vi "Write Last Temperature.vi"(8 "error in (no error)":errorcluster, 10 "Last Temperature":dbl format="%#_g °C", 11 "Thermometer Base in":refnum<class "Thermometer Base.lvclass">) -> (0 "error out":errorcluster, 3 "Thermometer Base out":refnum<class "Thermometer Base.lvclass">)   [LabVIEW 2023, in "Thermometer.lvlib" / "Thermometer Base.lvlib" / "Thermometer Base.lvclass"]
uses:
  Thermometer Base.lvclass
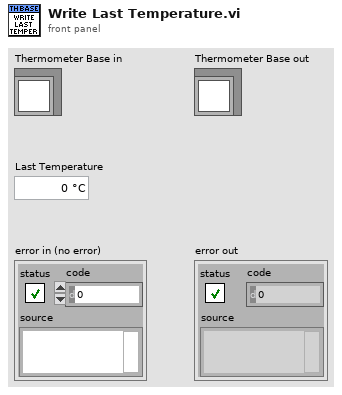
[diagram p1: front panel]
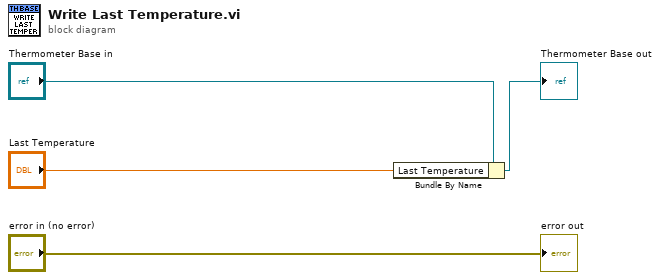
[diagram p0: block diagram]
diagram:
  n1 = Bundle By Name(cluster="Thermometer Base in", "Last Temperature"="Last Temperature") -> (→"Thermometer Base out":refnum<class "Thermometer Base.lvclass">)
  "error out" <- "error in (no error)"
